vi "WriteToStdOut.vi"(7 "Refnum":u64, 8 "error in (no error)":errorcluster, 9 "TimeStamp":timestamp, 10 "Data":string, 11 "Cli in":refnum<class "Cli.lvclass">) -> (0 "error out":errorcluster, 3 "Cli out":refnum<class "Cli.lvclass">)   [LabVIEW 2022 SP3, in "Cli.lvlib" / "Cli.lvclass"]
uses:
  Cli.lvclass
  Tcp/Tcp Messages/ConnectionWriteData Msg/ConnectionWriteData Msg.lvclass
  Tcp/DataToSend/DataToSend.lvclass
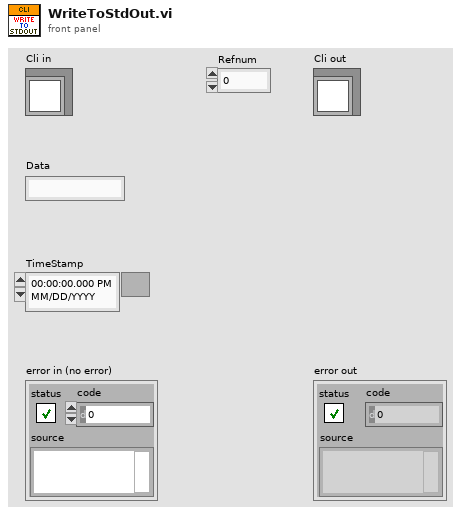
[diagram p1: front panel]
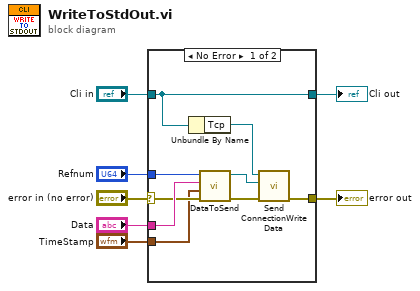
[diagram p0: block diagram]
diagram:
  n1 = case shown="No Error" "error in (no error)" {
    selector: "error in (no error)" -> [w14 w18]
    tunnel: [w12 w18] -> w6
    tunnel: [w10 w17] -> w4
    tunnel: "Cli in" -> [w10 w17]
    tunnel: "Refnum" -> [w16 _]
    tunnel: "Data" -> [w15 _]
    tunnel: "TimeStamp" -> [w8 _]
    frame No Error {
      n2 = Unbundle By Name(w10) -> ("Tcp"=w9:refnum<class "Message Enqueuer.lvclass">)
      n3 = call "DataToSend.vi"("error in (no error)"=w14, "TimeStamp"=w8, "Data"=w15, "Refnum"=w16) -> ("error out"=w13:errorcluster, "DataToSend"=w11:refnum<class "DataToSend.lvclass">)  [unwired: 6 in]
      n4 = call "Send ConnectionWriteData.vi"("error in (no error)"=w13, "DataToSend"=w11, "Message Enqueuer"=w9) -> ("error out"=w12:errorcluster)  [unwired: 7 in, 1 out]
    }
    frame Error {
    }
  }
  "error out" <- w6
  "Cli out" <- w4
